vi "format endpoint termination.vi"(10 "Base URL":string="https://api.gov.nominal.io/api/") -> (2 "Base URL with /":string)   [LabVIEW 2020, in "Nominal Client.lvclass"]
uses:
  Nominal Client.lvclass
  Nominal Client.lvclass/Nominal Client.ctl
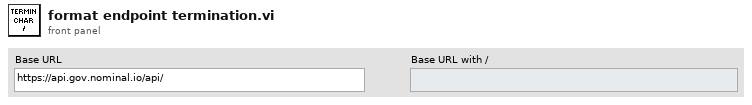
[diagram p1: front panel]
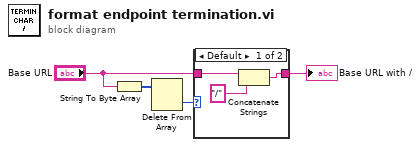
[diagram p0: block diagram]
diagram:
  n1 = String To Byte Array(string="Base URL") -> (unsigned byte array=w4:u8[])
  n2 = Delete From Array(array=w4) -> (deleted portion=w3:u8)  [unwired: 2 in, 1 out]
  n3 = case shown="Default" w3 {
    tunnel: "Base URL" -> [w7 w8]
    tunnel: [w6 w8] -> w1
    frame Default {
      n4 = Concatenate Strings(w7, "/" ("string")) -> (w6:string)
    }
    frame 47 {
    }
  }
  "Base URL with /" <- w1
